vi "NISE.remote.Set Generic Property (Core).vi"(0 "SLSC Remote in":refnum<class "SLSC Interface.lvclass">, 1 "property type":T1, 5 "resources":string="$DefaultDevices", 7 "property":refnum<k21>, 9 "property value":variant, 11 "error in (no error)":errorcluster) -> (4 "SLSC Remote out":refnum<class "SLSC Interface.lvclass">, 15 "error out":errorcluster)   [LabVIEW 2016, in "SLSC Interface.lvclass"]
uses:
  SLSC Interface Class/SLSC Interface.lvclass
  SLSC Interface Class/NISE.Property Type.ctl
  SLSC Interface Class/SLSC Interface.lvclass/SLSC Interface.ctl
  SLSC Interface Class/NISE.Read client handle.vi
  SLSC Interface Class/NISE.Read URL.vi
  SLSC Interface Class/NISE.Read session.vi
  <vilib>/NI/NI JSONRPC Server Framework/Classes/Server/server.Format Client Request (Auto-Increment).vi
  <vilib>/httpClient/POSTBuffer.vi
  <vilib>/httpClient/LabVIEWHTTPClient.lvlib
  <vilib>/NI/NI JSONRPC Server Framework/Classes/Server/JSONRPC Server.lvclass
  <vilib>/NI/JSON Support for LabVIEW/JSON Value/JSON Value.lvclass
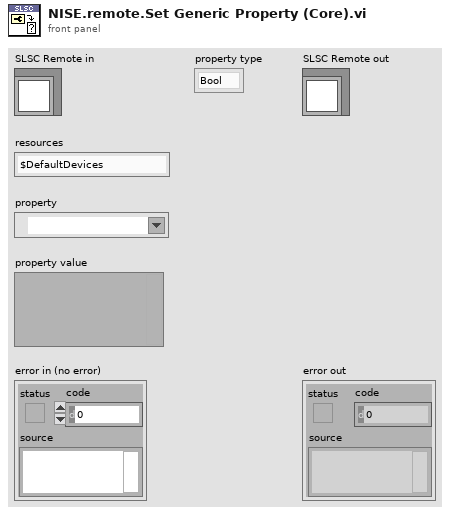
[diagram p1: front panel]
types:
  T1 = typedef "SLSC Interface.lvclass/NISE.Property Type.ctl" = enum16{"Bool", "DBL", "I32", "I64", "String", "U32", "U64", "1D Bool", "1D DBL", "1D I32", "1D I64", "1D String", "1D U32", "1D U64"}
  T2 = typedef "LabVIEWHTTPClient.lvlib/ClientHandle.ctl" = refnum<k1>
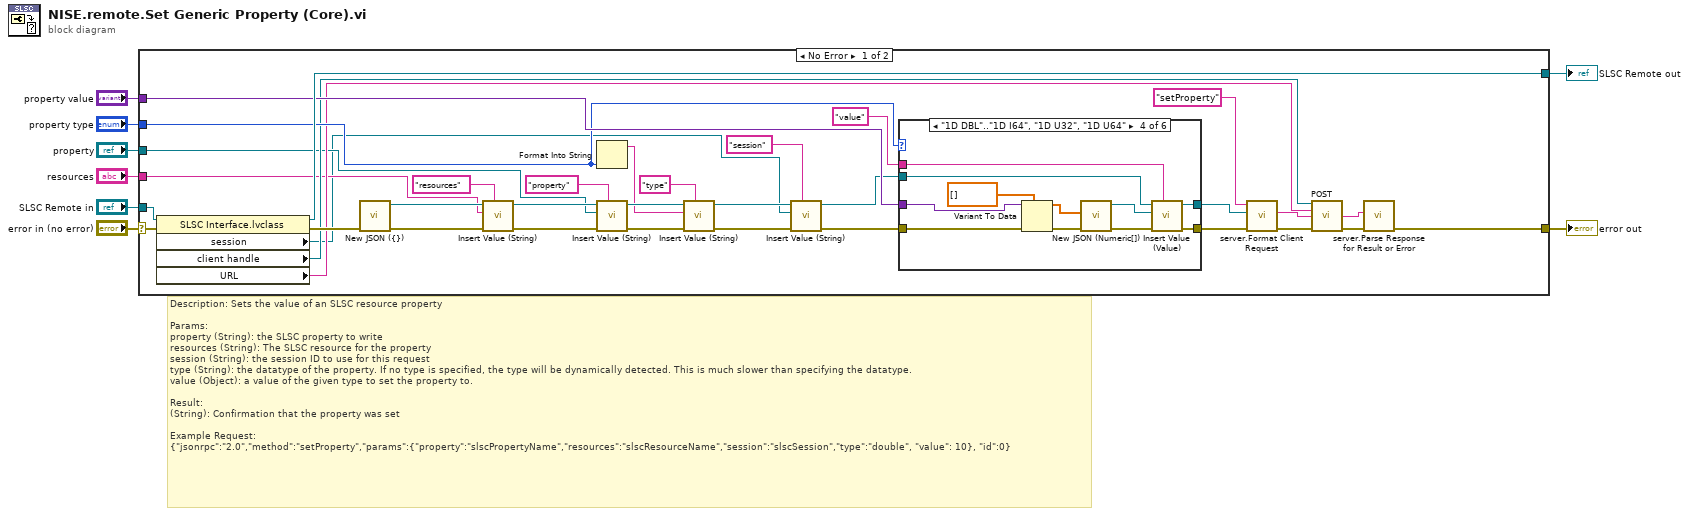
[diagram p0: block diagram]
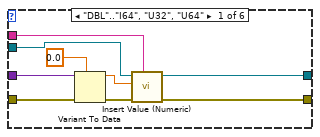
[diagram p2: hidden frame]
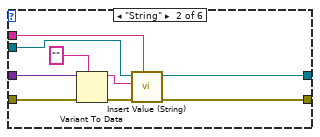
[diagram p3: hidden frame]
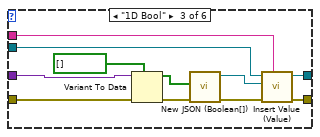
[diagram p4: hidden frame]
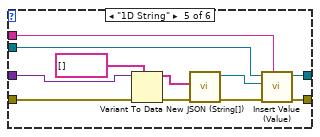
[diagram p5: hidden frame]
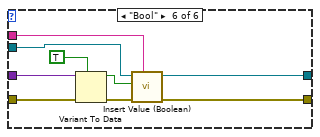
[diagram p6: hidden frame]
diagram:
  # "Description: Sets the value of an SLSC resource property\n\nParams:\nproperty (String): the SLSC property to write\nresources (String): The SLSC resource for the property\nsession (String): the session ID to use for this request\ntype (String): the datatype of the property. If no type is specified, the type will be dynamically detected. This is much slower than specifying the datatype.\nvalue (Object): a value of the given type to set the property to.\n\nResult:\n(String): Confirmation that the property was set\n\nExample Request: \n{\"jsonrpc\":\"2.0\",\"method\":\"setProperty\",\"params\":{\"property\":\"slscPropertyName\",\"resources\":\"slscResourceName\",\"session\":\"slscSession\",\"type\":\"double\", \"value\": 10}, \"id\":0}"
  n1 = case shown="No Error" "error in (no error)" {
    selector: "error in (no error)" -> [w39 w104]
    tunnel: "resources" -> [w10 _]
    tunnel: "SLSC Remote in" -> [w43 w105]
    tunnel: [w42 w105] -> w6
    tunnel: "property" -> [w11 _]
    tunnel: "property value" -> [w41 _]
    tunnel: "property type" -> [w35 _]
    tunnel: [w21 w104] -> w1
    frame No Error {
      n2 = property class="SLSC Interface.lvclass"(reference=w43, error in=w39) -> (reference out=w42:refnum<class "SLSC Interface.lvclass">, error out=w38:errorcluster, "session"=w9:refnum<k21>, "client handle"=w26:T2, "URL"=w25:string)
      n3 = call <vilib>:"New JSON ({}).vi"("error in (no error)"=w38) -> ("error out"=w37:errorcluster, "JSON Value out"=w16:refnum<class "JSON Value.lvclass">)  [unwired: 9 in]
      n4 = call <vilib>:"Insert Value (String).vi"("key"="resources" ("Name"), "error in (no error)"=w37, "value"=w10, "JSON Value in"=w16) -> ("error out"=w36:errorcluster, "JSON Value out"=w15:refnum<class "JSON Value.lvclass">)  [unwired: 5 in, 1 out]
      n5 = Format Into String(w35) -> (resulting string=w12:string)  [unwired: 3 in, 1 out]
      n6 = call <vilib>:"Insert Value (String).vi"("key"="property" ("Name"), "error in (no error)"=w36, "value"=w11, "JSON Value in"=w15) -> ("error out"=w32:errorcluster, "JSON Value out"=w14:refnum<class "JSON Value.lvclass">)  [unwired: 5 in, 1 out]
      n7 = call <vilib>:"Insert Value (String).vi"("key"="type" ("String"), "error in (no error)"=w32, "value"=w12, "JSON Value in"=w14) -> ("error out"=w31:errorcluster, "JSON Value out"=w13:refnum<class "JSON Value.lvclass">)  [unwired: 5 in, 1 out]
      n8 = call <vilib>:"Insert Value (String).vi"("key"="session" ("Name"), "error in (no error)"=w31, "value"=w9, "JSON Value in"=w13) -> ("error out"=w29:errorcluster, "JSON Value out"=w30:refnum<class "JSON Value.lvclass">)  [unwired: 5 in, 1 out]
      n9 = case shown="\"1D DBL\"..\"1D I64\", \"1D U32\", \"1D U64\"" w35 {
        tunnel: w41 -> [w52 w61 w72 w83 w94 w103]
        tunnel: "value" ("Name") -> [w45 w53 w65 w76 w92 w97]
        tunnel: w29 -> [w50 w59 w70 w81 w91 w101]
        tunnel: [w48 w57 w68 w79 w89 w99] -> w27
        tunnel: [w47 w56 w67 w78 w88 w98] -> w28
        tunnel: w30 -> [w44 w54 w66 w77 w84 w95]
        frame "DBL".."I64", "U32", "U64" {
          n10 = Variant To Data(error in=w50, type=0.0 ("Numeric"), Variant=w52) -> (data=w46:dbl, error out=w49:errorcluster)
          n11 = call <vilib>:"Insert Value (Numeric).vi"("key"=w45, "error in (no error)"=w49, "value"=w46, "JSON Value in"=w44) -> ("error out"=w47:errorcluster, "JSON Value out"=w48:refnum<class "JSON Value.lvclass">)  [unwired: 5 in, 1 out]
        }
        frame "String" {
          n12 = Variant To Data(error in=w59, type="" ("Numeric"), Variant=w61) -> (data=w55:string, error out=w58:errorcluster)
          n13 = call <vilib>:"Insert Value (String).vi"("key"=w53, "error in (no error)"=w58, "value"=w55, "JSON Value in"=w54) -> ("error out"=w56:errorcluster, "JSON Value out"=w57:refnum<class "JSON Value.lvclass">)  [unwired: 5 in, 1 out]
        }
        frame "1D Bool" {
          n14 = Variant To Data(error in=w70, type=bool[] [], Variant=w72) -> (data=w63:bool[], error out=w69:errorcluster)
          n15 = call <vilib>:"New JSON (Boolean[]).vi"("error in (no error)"=w69, "Boolean Array"=w63) -> ("error out"=w64:errorcluster, "JSON Value out"=w62:refnum<class "JSON Value.lvclass">)  [unwired: 8 in]
          n16 = call <vilib>:"Insert Value (Value).vi"("key"=w65, "error in (no error)"=w64, 10:"JSON Value in"=w62, 11:"JSON Value in"=w66) -> ("error out"=w67:errorcluster, "JSON Value out"=w68:refnum<class "JSON Value.lvclass">)  [unwired: 5 in, 1 out]
        }
        frame "1D DBL".."1D I64", "1D U32", "1D U64" {
          n17 = Variant To Data(error in=w81, type=dbl[] [], Variant=w83) -> (data=w74:dbl[], error out=w80:errorcluster)
          n18 = call <vilib>:"New JSON (Numeric[]).vi"("error in (no error)"=w80, "Numeric Array"=w74) -> ("error out"=w75:errorcluster, "JSON Value out"=w73:refnum<class "JSON Value.lvclass">)  [unwired: 8 in]
          n19 = call <vilib>:"Insert Value (Value).vi"("key"=w76, "error in (no error)"=w75, 10:"JSON Value in"=w73, 11:"JSON Value in"=w77) -> ("error out"=w78:errorcluster, "JSON Value out"=w79:refnum<class "JSON Value.lvclass">)  [unwired: 5 in, 1 out]
        }
        frame "1D String" {
          n20 = Variant To Data(error in=w91, type=string[] [], Variant=w94) -> (data=w86:string[], error out=w90:errorcluster)
          n21 = call <vilib>:"New JSON (String[]).vi"("error in (no error)"=w90, "String Array"=w86) -> ("error out"=w87:errorcluster, "JSON Value out"=w85:refnum<class "JSON Value.lvclass">)  [unwired: 8 in]
          n22 = call <vilib>:"Insert Value (Value).vi"("key"=w92, "error in (no error)"=w87, 10:"JSON Value in"=w85, 11:"JSON Value in"=w84) -> ("error out"=w88:errorcluster, "JSON Value out"=w89:refnum<class "JSON Value.lvclass">)  [unwired: 5 in, 1 out]
        }
        frame "Bool" {
          n23 = Variant To Data(error in=w101, type=TRUE, Variant=w103) -> (data=w96:bool, error out=w100:errorcluster)
          n24 = call <vilib>:"Insert Value (Boolean).vi"("key"=w97, "error in (no error)"=w100, "value"=w96, "JSON Value in"=w95) -> ("error out"=w98:errorcluster, "JSON Value out"=w99:refnum<class "JSON Value.lvclass">)  [unwired: 5 in, 1 out]
        }
      }
      n25 = call-poly <vilib>:"server.Format Client Request.vi"("error in (no error)"=w28, "JSON Value in"=w27, "method"="setProperty") -> ("error out"=w24:errorcluster, "Request String"=w33:string)  [unwired: 7 in]
      n26 = call-poly <vilib>:"POST.vi"("client handle"=w26, "url"=w25, "buffer"=w33, "error in (no error)"=w24) -> ("body"=w23:string, "error out"=w22:errorcluster)  [unwired: 8 in, 2 out]
      n27 = call <vilib>:"server.Parse Response for Result or Error.vi"("error in"=w22, "Response String In"=w23) -> ("error out"=w21:errorcluster)  [unwired: 7 in, 2 out]
    }
    frame Error {
    }
  }
  "error out" <- w1
  "SLSC Remote out" <- w6
